vi "Update View Event.vi"(6 "VIRef":refnum<vi>, 7 "Name":string, 8 "error in (no error)":errorcluster, 9 "Wight":u32=500, 10 "Height":u32=500, 11 "States Out":string) -> (0 "error out":errorcluster, 3 "Remaining States":string)   [LabVIEW 2020]
uses:
  MDI ViewManager/Typedef/Update View.ctl
  ea4809dd-d388-4c33-a745-4070a3c47c80.vi
  <userlib>/_NEVSTOP/Communicable State Machine(CSM)/AdvanceAPI/CSM - Break Down Multiple States String.vi
  <userlib>/_NEVSTOP/Communicable State Machine(CSM)/AdvanceAPI/CSM - Compact Multiple States.vi
  <userlib>/_NEVSTOP/Communicable State Machine(CSM)/addons/API-String-Arugments-Support/_Support/Data To API String Arguments.vi
  <userlib>/_NEVSTOP/Communicable State Machine(CSM)/Communicable State Machine.lvlib
  MDI ViewManager/MDI ViewManager.lvlib
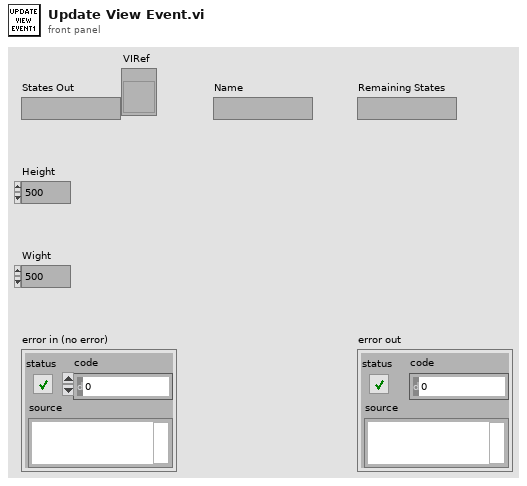
[diagram p1: front panel]
types:
  T1 = typedef "MDI ViewManager.lvlib/Update View.ctl" = cluster{"Name":string, "VIPath":path, "Height(Default)":u32, "Widht(Default)":u32, "VIRef":refnum<vi>}
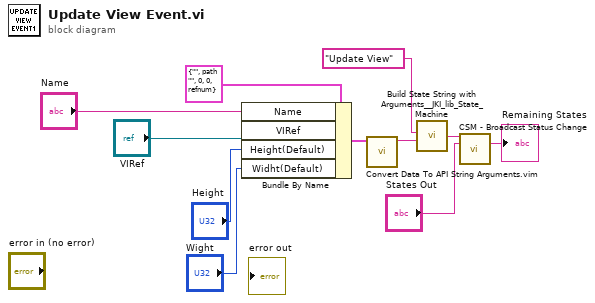
[diagram p0: block diagram]
diagram:
  n1 = Bundle By Name(cluster=T1 {"Name"="", "VIPath"=path "", "Height(Default)"=0, "Widht(Default)"=0, "VIRef"=refnum} ("value"), "Name"="Name", "VIRef"="VIRef", "Height(Default)"="Height", "Widht(Default)"="Wight") -> (w6:T1)
  n2 = call "Convert Data To API String Arguments.vim"("Data"=w6) -> ("API String"=w5:string)  [unwired: 7 in, 1 out]
  n3 = call <vilib>:"Build State String with Arguments__JKI_lib_State_Machine.vi"("Arguments (\"\")"=w5, "State"="Update View" ("Status With Arguments")) -> ("State with Arguments"=w11:string)  [unwired: 4 in]
  n4 = call <userlib>:"CSM - Broadcast Status Change.vi"("Status With Arguments"=w11, "State Queue"="States Out") -> ("Remaining States"=→"Remaining States":string)  [unwired: 13 in]
